vi "BME_DG_DetectOnPCIBus.vi"(8 "error in (no error)":errorcluster, 9 "p_Error in":i32) -> (0 "error out":errorcluster, 3 "NumberOfCards":i32)   [LabVIEW 2009, in "POLARIS BME DG.lvlib"]
uses:
  POLARIS BME DG.lvlib
  BME DLL/DelayGenerator.dll
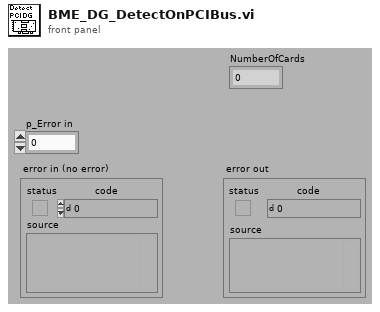
[diagram p1: front panel]
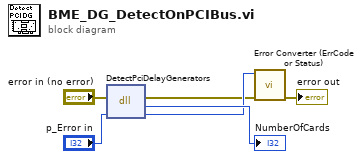
[diagram p0: block diagram]
diagram:
  n1 = dll-call lib="C:/CS Framework/LVSCC/LV2009/GPL/Projects/cs-framework/CSClass/CSPOLARIS/POLARIS BME DG/BME DLL/DelayGenerator.dll" fn="DetectPciDelayGenerators"(error in="error in (no error)", "p_Error"="p_Error in") -> (error out=w2:errorcluster, "NumberOfCards"=→"NumberOfCards":i32, "p_Error"=w3:i32)  [unwired: 2 in, 1 out]
  n2 = call "Error Converter (ErrCode or Status).vi"("error in (no error)"=w2, "error code"=w3) -> ("error out"=→"error out":errorcluster)  [unwired: 9 in]
